vi "test_F9P.vi"() -> ()   [LabVIEW 2019] (continued)
3*05\r\n$GNGSA,A,3,28,11,14,13,33,08,10,,,,,,1.09,0.62,0.90,4*05\r\n$GPGSV,4,1,13,02,65,334,46,04,08,037,34,05,48,261,21,06,58,076,43,1*69\r\n$GPGSV,4,2,13,07,06,105,26,09,38,057,45,12,18,263,29,13,08,191,21,1*66\r\n$GPGSV,4,3,13,17,19,158,23,19,37,161,24,25,11,294,,29,07,323,20,1*6A\r\n$GPGSV,4,4,13,30,01,134,,1*52\r\n$GPGSV,4,1,13,02,65,334,,04,08,037,19,05,48,261,30,06,58,076,31,6*66\r\n$GPGSV,4,2,13,07,06,105,,09,38,057,39,12,18,263,,13,08,191,,6*66\r\n$GPGSV,4,3,13,17,19,158,24,19,37,161,,25,11,294,,29,07,323,,6*6E\r\n$GPGSV,4,4,13,30,01,134,,6*55\r\n$GLGSV,2,1,06,70,54,030,36,71,69,224,32,72,18,217,37,84,08,134,09,1*76\r\n$GLGSV,2,2,06,85,63,113,40,86,52,337,,1*7F\r\n$GLGSV,2,1,06,70,54,030,,71,69,224,17,72,18,217,26,84,08,134,15,3*7B\r\n$GLGSV,2,2,06,85,63,113,24,86,52,337,,3*7F\r\n$GAGSV,3,1,09,02,04,287,07,04,68,085,40,09,44,196,29,11,78,037,39,7*7A\r\n$GAGSV,3,2,09,12,32,115,31,18,55,284,29,19,17,042,20,25,01,241,,7*79\r\n$GAGSV,3,3,09,36,35,314,37,7*4B\r\n$GAGSV,3,1,09,02,04,287,,04,68,085,36,09,44,196,33,11,78,037,28,2*72\r\n$GAGSV,3,2,09,12,32,115,27,18,55,284,38,19,17,042,33,25,01,241,,2*79\r\n$GAGSV,3,3,09,36,35,314,23,2*4B\r\n$GBGSV,4,1,13,04,35,133,,05,09,257,,06,27,182,,07,09,201,,1*7B\r\n$GBGSV,4,2,13,08,65,355,41,09,07,194,,10,16,222,18,11,37,142,22,1*73\r\n$GBGSV,4,3,13,13,50,315,42,14,76,037,41,28,59,310,42,33,73,239,15,1*7A\r\n$GBGSV,4,4,13,34,13,142,17,1*40\r\n$GBGSV,4,1,13,04,35,133,,05,09,257,,06,27,182,,07,09,201,16,3*7E\r\n$GBGSV,4,2,13,08,65,355,35,09,07,194,,10,16,222,27,11,37,142,32,3*7F\r\n$GBGSV,4,3,13,13,50,315,40,14,76,037,28,28,59,310,,33,73,239,,3*77\r\n$GBGSV,4,4,13,34,13,142,,3*44\r\n$GNGLL,3723.61676,N,12656.96910,E,064321.00,A,A*71\r\n$GNRMC,064322.00,A,3723.61692,N,12656.96920,E,0.256,,250720,,,A,V*1B\r\n$GNVTG,,T,,M,0.256,N,0.474,K,A*3B\r\n$GNGGA,064322.00,3723.61692,N,12656.96920,E,1,12,0.62,44.9,M,18.5,M,,*7C\r\n$GNGSA,A,3,17,19,06,05,02,12,09,,,,,,1.07,0.62,0.87,1*09\r\n$GNGSA,A,3,85,70,71,72,,,,,,,,,1.07,0.62,0.87,2*06\r\n$GNGSA,A,3,36,19,11,04,09,12,,,,,,,1.07,0.62,0.87,3*0D\r\n$GNGSA,A,3,28,14,13,33,08,10,,,,,,,1.07,0.62,0.87,4*0D\r\n$GPGSV,4,1,13,02,65,334,45,04,08,037,35,05,48,261,30,06,58,076,44,1*6C\r\n$GPGSV,4,2,13,07,06,105,25,09,38,057,44,12,18,263,28,13,08,191,20,1*64\r\n$GPGSV,4,3,13,17,19,158,30,19,37,161,31,25,11,294,,29,07,323,20,1*6C\r\n$GPGSV,4,4,13,30,01,134,,1*52\r\n$GPGSV,4,1,13,02,65,334,,04,08,037,19,05,48,261,34,06,58,076,33,6*60\r\n$GPGSV,4,2,13,07,06,105,,09,38,057,41,12,18,263,,13,08,191,,6*69\r\n$GPGSV,4,3,13,17,19,158,24,19,37,161,,25,11,294,,29,07,323,,6*6E\r\n$GPGSV,4,4,13,30,01,134,,6*55\r\n$GLGSV,2,1,06,70,54,030,36,71,69,224,31,72,18,217,41,84,08,134,12,1*7E\r\n$GLGSV,2,2,06,85,63,113,39,86,52,337,,1*71\r\n$GLGSV,2,1,06,70,54,030,,71,69,224,17,72,18,217,26,84,08,134,18,3*76\r\n$GLGSV,2,2,06,85,63,113,23,86,52,337,,3*78\r\n$GAGSV,3,1,09,02,04,287,09,04,68,085,41,09,44,196,36,11,78,037,39,7*7B\r\n$GAGSV,3,2,09,12,32,115,35,18,55,284,24,19,17,042,30,25,01,241,,7*71\r\n$GAGSV,3,3,09,36,35,314,35,7*49\r\n$GAGSV,3,1,09,02,04,287,,04,68,085,36,09,44,196,33,11,78,037,28,2*72\r\n$GAGSV,3,2,09,12,32,115,27,18,55,284,37,19,17,042,28,25,01,241,,2*7C\r\n$GAGSV,3,3,09,36,35,314,23,2*4B\r\n$GBGSV,4,1,13,04,35,133,,05,09,257,,06,27,182,,07,09,201,,1*7B\r\n$GBGSV,4,2,13,08,65,355,41,09,07,194,,10,16,222,17,11,37,142,24,1*7A\r\n$GBGSV,4,3,13,13,50,315,42,14,76,037,41,28,59,310,42,33,73,239,27,1*7B\r\n$GBGSV,4,4,13,34,13,142,17,1*40\r\n$GBGSV,4,1,13,04,35,133,,05,09,257,,06,27,182,,07,09,201,16,3*7E\r\n$GBGSV,4,2,13,08,65,355,31,09,07,194,,10,16,222,27,11,37,142,,3*7A\r\n$GBGSV,4,3,13,13,50,315,40,14,76,037,36,28,59,310,,33,73,239,,3*78\r\n$GBGSV,4,4,13,34,13,142,,3*44\r\n$GNGLL,3723.61692,N,12656.96920,E,064322.00,A,A*7B\r\n$GNRMC,064323.00,A,3723.61711,N,12656.96949,E,1.226,107.58,250720,,,A,V*0C\r\n$GNVTG,107.58,T,,M,1.226,N,2.271,K,A*29\r\n$GNGGA,064323.00,3723.61711,N,12656.96949,E,1,12,0.62,44.9,M,18.5,M,,*78\r\n$GNGSA,A,3,17,19,06,05,02,12,09,,,,,,1.09,0.62,0.90,1*01\r\n$GNGSA,A,3,85,70,71,72,,,,,,,,,1.09,0.62,0.90,2*0E\r\n$GNGSA,A,3,36,19,11,04,09,12,,,,,,,1.09,0.62,0.90,3*05\r\n$GNGSA,A,3,28,11,14,13,33,08,10,,,,,,1.09,0.62,0.90,4*05\r\n$GPGSV,4,1,13,02,65,334,44,04,08,037,37,05,48,261,36,06,58,076,46,1*6B\r\n$GPGSV,4,2,13,07,06,105,24,09,38,057,44,12,18,263,27,13,08,191,18,1*61\r\n$GPGSV,4,3,13,17,19,158,29,19,37,161,30,25,11,294,,29,07,323,19,1*6F\r\n$GPGSV,4,4,13,30,01,134,,1*52\r\n$GPGSV,4,1,13,02,65,334,,04,08,037,28,05,48,261,35,06,58,076,36,6*66\r\n$GPGSV,4,2,13,07,06,105,,09,38,057,38,12,18,263,,13,08,191,,6*67\r\n$GPGSV,4,3,13,17,19,158,22,19,37,161,,25,11,294,,29,07,323,,6*68\r\n$GPGSV,4,4,13,30,01,134,,6*55\r\n$GLGSV,2,1,06,70,54,030,33,71,69,224,33,72,18,217,38,84,08,134,11,1*74\r\n$GLGSV,2,2,06,85,63,113,35,86,52,337,,1*7D\r\n$GLGSV,2,1,06,70,54,030,,71,69,224,18,72,18,217,26,84,08,134,15,3*74\r\n$GLGSV,2,2,06,85,63,113,22,86,52,337,,3*79\r\n$GAGSV,3,1,09,02,04,287,12,04,68,085,38,09,44,196,32,11,78,037,37,7*75\r\n$GAGSV,3,2,09,12,32,115,32,18,55,284,26,19,17,042,34,25,01,241,,7*70\r\n$GAGSV,3,3,09,36,35,314,27,7*4A\r\n$GAGSV,3,1,09,02,04,287,,04,68,085,31,09,44,196,32,11,78,037,33,2*7E\r\n$GAGSV,3,2,09,12,32,115,33,18,55,284,35,19,17,042,32,25,01,241,,2*70\r\n$GAGSV,3,3,09,36,35,314,23,2*4B\r\n$GBGSV,4,1,13,04,35,133,,05,09,257,,06,27,182,,07,09,201,,1*7B\r\n$GBGSV,4,2,13,08,65,355,41,09,07,194,,10,16,222,15,11,37,142,31,1*7C\r\n$GBGSV,4,3,13,13,50,315,42,14,76,037,42,28,59,310,44,33,73,239,35,1*7D\r\n$GBGSV,4,4,13,34,13,142,20,1*44\r\n$GBGSV,4,1,13,04,35,133,,05,09,257,,06,27,182,,07,09,201,17,3*7F\r\n$GBGSV,4,2,13,08,65,355,34,09,07,194,,10,16,222,24,11,37,142,,3*7C\r\n$GBGSV,4,3,13,13,50,315,41,14,76,037,41,28,59,310,,33,73,239,,3*79\r\n$GBGSV,4,4,13,34,13,142,,3*44\r\n$GNGLL,3723.61711,N,12656.96949,E,064323.00,A,A*7F\r\n$GNRMC,064324.00,A,3723.61742,N,12656.97004,E,2.052,73.76,250720,,,A,V*30\r\n$GNVTG,73.76,T,,M,2.052,N,3.800,K,A*18\r\n$GNGGA,064324.00,3723.61742,N,12656.97004,E,1,12,0.66,44.7,M,18.5,M,,*72\r\n$GNGSA,A,3,17,19,06,05,02,09,,,,,,,1.18,0.66,0.98,1*0E\r\n$GNGSA,A,3,85,70,71,72,,,,,,,,,1.18,0.66,0.98,2*02\r\n$GNGSA,A,3,36,19,11,04,09,12,,,,,,,1.18,0.66,0.98,3*09\r\n$GNGSA,A,3,28,11,14,13,34,33,08,10,,,,,1.18,0.66,0.98,4*0E\r\n$GPGSV,4,1,13,02,65,334,46,04,08,037,37,05,48,261,37,06,58,076,37,1*6E\r\n$GPGSV,4,2,13,07,06,105,31,09,38,057,43,12,18,263,,13,08,191,,1*6E\r\n$GPGSV,4,3,13,17,19,158,22,19,37,161,34,25,11,294,25,29,07,323,18,1*66\r\n$GPGSV,4,4,13,30,01,134,,1*52\r\n$GPGSV,4,1,13,02,65,334,,04,08,037,38,05,48,261,36,06,58,076,37,6*65\r\n$GPGSV,4,2,13,07,06,105,,09,38,057,41,12,18,263,,13,08,191,,6*69\r\n$GPGSV,4,3,13,17,19,158,20,19,37,161,,25,11,294,,29,07,323,,6*6A\r\n$GPGSV,4,4,13,30,01,134,,6*55\r\n$GLGSV,2,1,06,70,54,030,38,71,69,224,37,72,18,217,34,84,08,134,12,1*74\r\n$GLGSV,2,2,06,85,63,113,29,86,52,337,,1*70\r\n$GLGSV,2,1,06,70,54,030,,71,69,224,32,72,18,217,27,84,08,134,14,3*7C\r\n$GLGSV,2,2,06,85,63,113,30,86,52,337,,3*7A\r\n$GAGSV,3,1,09,02,04,287,11,04,68,085,35,09,44,196,26,11,78,037,39,7*70\r\n$GAGSV,3,2,09,12,32,115,28,18,55,284,37,19,17,042,35,25,01,241,,7*7A\r\n$GAGSV,3,3,09,36,35,314,26,7*4B\r\n$GAGSV,3,1,09,02,04,287,,04,68,085,32,09,44,196,26,11,78,037,27,2*7D\r\n$GAGSV,3,2,09,12,32,115,29,18,55,284,38,19,17,042,36,25,01,241,,2*72\r\n$GAGSV,3,3,09,36,35,314,23,2*4B\r\n$GBGSV,4,1,13,04,35,133,,05,09,257,,06,27,182,,07,09,201,,1*7B\r\n$GBGSV,4,2,13,08,65,355,42,09,07,194,,10,16,222,15,11,37,142,32,1*7C\r\n$GBGSV,4,3,13,13,50,315,43,14,76,037,42,28,59,310,43,33,73,239,39,1*77\r\n$GBGSV,4,4,13,34,13,142,22,1*46\r\n$GBGSV,4,1,13,04,35,133,,05,09,257,,06,27,182,,07,09,201,19,3*71\r\n$GBGSV,4,2,13,08,65,355,36,09,07,194,,10,16,222,21,11,37,142,,3*7B\r\n$GBGSV,4,3,13,13,50,315,39,14,76,037,33,28,59,310,,33,73,239,,3*73\r\n$GBGSV,4,4,13,34,13,142,,3*44\r\n$GNGLL,3723.61742,N,12656.97004,E,064324.00,A,A*7F\r\n$GNRMC,064325.00,A,3723.61775,N,12656.97077,E,2.478,66.36,250720,,,A,V*3D\r\n$GNVTG,66.36,T,,M,2.478,N,4.589,K,A*1F\r\n$GNGGA,064325.00,3723.61775,N,12656.97077,E,1,12,0.66,44.5,M,18.5,M,,*71\r\n$GNGSA,A,3,17,19,06,05,02,09,,,,,,,1.18,0.66,0.98,1*0E\r\n$GNGSA,A,3,85,70,71,72,,,,,,,,,1.18,0.66,0.98,2*02\r\n$GNGSA,A,3,36,19,11,04,09,12,,,,,,,1.18,0.66,0.98,3*09\r\n$GNGSA,A,3,28,11,14,13,33,08,10,,,,,,1.18,0.66,0.98,4*09\r\n$GPGSV,4,1,13,02,66,335,48,04,08,037,36,05,48,261,33,06,58,076,42,1*65\r\n$GPGSV,4,2,13,07,06,105,,09,38,057,45,12,18,263,,13,08,191,,1*6A\r\n$GPGSV,4,3,13,17,19,158,25,19,37,161,36,25,11,294,22,29,07,323,18,1*64\r\n$GPGSV,4,4,13,30,01,134,,1*52\r\n$GPGSV,4,1,13,02,66,335,,04,08,037,40,05,48,261,38,06,58,076,36,6*67\r\n$GPGSV,4,2,13,07,06,105,,09,38,057,35,12,18,263,22,13,08,191,,6*6A\r\n$GPGSV,4,3,13,17,19,158,20,19,37,161,,25,11,294,,29,07,323,,6*6A\r\n$GPGSV,4,4,13,30,01,134,,6*55\r\n$GLGSV,2,1,06,70,54,030,39,71,69,224,35,72,18,217,32,84,08,134,09,1*7B\r\n$GLGSV,2,2,06,85,63,113,34,86,52,337,,1*7C\r\n$GLGSV,2,1,06,70,54,030,,71,69,224,26,72,18,217,27,84,08,134,15,3*78\r\n$GLGSV,2,2,06,85,63,113,28,86,52,337,,3*73\r\n$GAGSV,3,1,09,02,04,287,09,04,68,085,36,09,44,196,32,11,78,037,39,7*7F\r\n$GAGSV,3,2,09,12,32,115,32,18,55,284,36,19,17,042,35,25,01,241,,7*70\r\n$GAGSV,3,3,09,36,35,314,26,7*4B\r\n$GAGSV,3,1,09,02,04,287,,04,68,085,31,09,44,196,26,11,78,037,32,2*7A\r\n$GAGSV,3,2,09,12,32,115,28,18,55,284,39,19,17,042,36,25,01,241,,2*72\r\n$GAGSV,3,3,09,36,35,314,22,2*4A\r\n$GBGSV,4,1,13,04,35,133,,05,09,257,,06,27,182,,07,09,201,,1*7B\r\n$GBGSV,4,2,13,08,65,355,41,09,07,194,,10,16,222,15,11,37,142,27,1*7B\r\n$GBGSV,4,3,13,13,50,315,45,14,76,037,41,28,59,310,44,33,73,239,38,1*74\r\n$GBGSV,4,4,13,34,13,142,,1*46\r\n$GBGSV,4,1,13,04,35,133,,05,09,257,,06,27,182,,07,09,201,20,3*7B\r\n$GBGSV,4,2,13,08,65,355,38,09,07,194,,10,16,222,18,11,37,142,,3*7F\r\n$GBGSV,4,3,13,13,50,315,40,14,76,037,34,28,59,310,,33,73,239,,3*7A\r\n$GBGSV,4,4,13,34,13,142,,3*44\r\n$GNGLL,3723.61775,N,12656.97077,E,064325.00,A,A*7E\r\n$GNRMC,064326.00,A,3723.61798,N,12656.97166,E,2.758,70.76,250720,,,A,V*3E\r\n$GNVTG,70.76,T,,M,2.758,N,5.109,K,A*10\r\n$GNGGA,064326.00,3723.61798,N,12656.97166,E,1,12,0.66,44.4,M,18.5,M,,*71\r\n$GNGSA,A,3,17,19,06,05,02,09,,,,,,,1.18,0.66,0.98,1*0E\r\n$GNGSA,A,3,85,70,71,72,,,,,,,,,1.18,0.66,0.98,2*02\r\n$GNGSA,A,3,36,19,11,04,09,12,,,,,,,1.18,0.66,0.98,3*09\r\n$GNGSA,A,3,28,11,14,13,33,08,10,,,,,,1.18,0.66,0.98,4*09\r\n$GPGSV,4,1,13,02,66,335,46,04,08,037,42,05,48,261,36,06,58,076,43,1*6C\r\n$GPGSV,4,2,13,07,06,105,,09,38,057,44,12,18,263,23,13,08,191,25,1*6D\r\n$GPGSV,4,3,13,17,19,158,25,19,37,161,36,25,11,294,20,29,07,323,19,1*67\r\n$GPGSV,4,4,13,30,01,134,,1*52\r\n$GPGSV,4,1,13,02,66,335,,04,08,037,39,05,48,261,40,06,58,076,35,6*65\r\n$GPGSV,4,2,13,07,06,105,,09,38,057,38,12,18,263,19,13,08,191,,6*6F\r\n$GPGSV,4,3,13,17,19,158,28,19,37,161,,25,11,294,,29,07,323,,6*62\r\n$GPGSV,4,4,13,30,01,134,,6*55\r\n$GLGSV,2,1,06,70,54,030,34,71,69,224,39,72,18,217,32,84,08,134,12,1*70\r\n$GLGSV,2,2,06,85,63,113,35,86,52,337,,1*7D\r\n$GLGSV,2,1,06,70,54,030,,71,69,224,26,72,18,217,25,84,08,134,16,3*79\r\n$GLGSV,2,2,06,85,63,113,27,86,52,337,,3*7C\r\n$GAGSV,3,1,09,02,04,287,12,04,68,085,41,09,44,196,26,11,78,037,39,7*70\r\n$GAGSV,3,2,09,12,32,115,28,18,55,284,39,19,17,042,35,25,01,241,,7*74\r\n$GAGSV,3,3,09,36,35,314,25,7*48\r\n$GAGSV,3,1,09,02,04,287,,04,68,085,32,09,44,196,23,11,78,037,32,2*7C\r\n$GAGSV,3,2,09,12,32,115,33,18,55,284,37,19,17,042,28,25,01,241,,2*79\r\n$GAGSV,3,3,09,36,35,314,21,2*49\r\n$GBGSV,4,1,13,04,35,133,,05,09,257,,06,27,182,,07,09,201,,1*7B\r\n$GBGSV,4,2,13,08,65,355,42,09,07,194,,10,16,222,17,11,37,142,31,1*7D\r\n$GBGSV,4,3,13,13,50,315,45,14,76,037,44,28,59,310,36,33,73,239,42,1*79\r\n$GBGSV,4,4,13,34,13,142,,1*46\r\n$GBGSV,4,1,13,04,35,133,,05,09,257,,06,27,182,,07,09,201,21,3*7A\r\n$GBGSV,4,2,13,08,65,355,38,09,07,194,,10,16,222,20,11,37,142,,3*74\r\n$GBGSV,4,3,13,13,50,315,40,14,76,037,38,28,59,310,,33,73,239,,3*76\r\n$GBGSV,4,4,13,34,13,142,,3*44\r\n$GNGLL,3723.61798,N,12656.97166,E,064326.00,A,A*7F\r\n$GNRMC,064327.00,A,3723.61827,N,12656.97258,E,2.933,66.94,250720,,,A,V*32\r\n$GNVTG,66.94,T,,M,2.933,N,5.432,K,A*15\r\n$GNGGA,064327.00,3723.61827,N,12656.97258,E,1,12,0.66,44.5,M,18.5,M,,*74\r\n$GNGSA,A,3,17,19,06,05,02,09,,,,,,,1.18,0.66,0.98,1*0E\r\n$GNGSA,A,3,85,70,71,72,,,,,,,,,1.18,0.66,0.98,2*02\r\n$GNGSA,A,3,36,19,11,04,09,12,,,,,,,1.18,0.66,0.98,3*09\r\n$GNGSA,A,3,28,11,14,13,33,34,08,10,,,,,1.18,0.66,0.98,4*0E\r\n$GPGSV,4,1,13,02,66,335,42,04,08,037,42,05,48,261,41,06,58,076,44,1*6F\r\n$GPGSV,4,2,13,07,06,105,,09,38,057,48,12,18,263,,13,08,191,25,1*60\r\n$GPGSV,4,3,13,17,19,158,27,19,37,161,32,25,11,294,18,29,07,323,17,1*64\r\n$GPGSV,4,4,13,30,01,134,,1*52\r\n$GPGSV,4,1,13,02,66,335,,04,08,037,35,05,48,261,37,06,58,076,37,6*6B\r\n$GPGSV,4,2,13,07,06,105,,09,38,057,40,12,18,263,13,13,08,191,,6*6A\r\n$GPGSV,4,3,13,17,19,158,25,19,37,161,,25,11,294,,29,07,323,,6*6F\r\n$GPGSV,4,4,13,30,01,134,,6*55\r\n$GLGSV,2,1,06,70,54,030,31,71,69,224,40,72,18,217,32,84,08,134,14,1*7D\r\n$GLGSV,2,2,06,85,63,113,33,86,52,337,,1*7B\r\n$GLGSV,2,1,06,70,54,030,,71,69,224,26,72,18,217,23,84,08,134,14,3*7D\r\n$GLGSV,2,2,06,85,63,113,26,86,52,337,,3*7D\r\n$GAGSV,3,1,09,02,04,287,08,04,68,085,43,09,44,196,27,11,78,037,39,7*78\r\n$GAGSV,3,2,09,12,32,115,28,18,55,284,38,19,17,042,37,25,01,241,,7*77\r\n$GAGSV,3,3,09,36,35,314,31,7*4D\r\n$GAGSV,3,1,09,02,04,287,,04,68,085,36,09,44,196,22,11,78,037,32,2*79\r\n$GAGSV,3,2,09,12,32,115,28,18,55,284,42,19,17,042,38,25,01,241,,2*70\r\n$GAGSV,3,3,09,36,35,314,23,2*4B\r\n$GBGSV,4,1,13,04,35,133,,05,09,257,,06,27,182,,07,09,201,,1*7B\r\n$GBGSV,4,2,13,08,65,355,42,09,07,194,,10,16,222,17,11,37,142,27,1*7A\r\n$GBGSV,4,3,13,13,50,315,37,14,76,037,44,28,59,310,42,33,73,239,40,1*7D\r\n$GBGSV,4,4,13,34,13,142,33,1*46\r\n$GBGSV,4,1,13,04,35,133,,05,09,257,,06,27,182,,07,09,201,23,3*78\r\n$GBGSV,4,2,13,08,65,355,36,09,07,194,,10,16,222,21,11,37,142,,3*7B\r\n$GBGSV,4,3,13,13,50,315,34,14,76,037,35,28,59,310,,33,73,239,,3*78\r\n$GBGSV,4,4,13,34,13,142,,3*44\r\n$GNGLL,3723.61827,N,12656.97258,E,064327.00,A,A*7B\r\n$GNRMC,064328.00,A,3723.61847,N,12656.97349,E,2.893,70.77,250720,,,A,V*3B\r\n$GNVTG,70.77,T,,M,2.893,N,5.358,K,A*1F\r\n$GNGGA,064328.00,3723.61847,N,12656.97349,E,1,12,0.66,44.2,M,18.5,M,,*7B\r\n$GNGSA,A,3,17,19,06,05,02,09,,,,,,,1.18,0.66,0.98,1*0E\r\n$GNGSA,A,3,85,70,71,72,,,,,,,,,1.18,0.66,0.98,2*02\r\n$GNGSA,A,3,36,19,11,04,09,12,,,,,,,1.18,0.66,0.98,3*09\r\n$GNGSA,A,3,28,11,14,13,33,08,10,,,,,,1.18,0.66,0.98,4*09\r\n$GPGSV,4,1,13,02,66,335,45,04,08,037,38,05,48,262,42,06,58,076,43,1*62\r\n$GPGSV,4,2,13,07,06,105,,09,38,057,47,12,18,263,,13,08,191,,1*68\r\n$GPGSV,4,3,13,17,19,158,31,19,37,161,28,25,11,294,18,29,07,323,17,1*68\r\n$GPGSV,4,4,13,30,01,134,,1*52\r\n$GPGSV,4,1,13,02,66,335,,04,08,037,36,05,48,262,39,06,58,076,33,6*61\r\n$GPGSV,4,2,13,07,06,105,,09,38,057,41,12,18,263,12,13,08,191,,6*6A\r\n$GPGSV,4,3,13,17,19,158,25,19,37,161,,25,11,294,,29,07,323,,6*6F\r\n$GPGSV,4,4,13,30,01,134,,6*55\r\n$GLGSV,2,1,06,70,54,030,35,71,69,224,39,72,18,217,27,84,08,134,11,1*76\r\n$GLGSV,2,2,06,85,63,113,35,86,52,337,,1*7D\r\n$GLGSV,2,1,06,70,54,030,,71,69,224,27,72,18,217,21,84,08,134,14,3*7E\r\n$GLGSV,2,2,06,85,63,113,27,86,52,337,,3*7C\r\n$GAGSV,3,1,09,02,04,287,10,04,68,085,41,09,44,196,26,11,78,037,39,7*72\r\n$GAGSV,3,2,09,12,32,115,29,18,55,284,39,19,17,042,42,25,01,241,,7*75\r\n$GAGSV,3,3,09,36,35,314,25,7*48\r\n$GAGSV,3,1,09,02,04,287,,04,68,085,33,09,44,196,22,11,78,037,31,2*7F\r\n$GAGSV,3,2,09,12,32,115,27,18,55,284,40,19,17,042,37,25,01,241,,2*72\r\n$GAGSV,3,3,09,36,35,314,24,2*4C\r\n$GBGSV,4,1,13,04,35,133,,05,09,257,,06,27,182,,07,09,201,,1*7B\r\n$GBGSV,4,2,13,08,65,355,42,09,07,194,,10,16,222,18,11,37,142,28,1*7A\r\n$GBGSV,4,3,13,13,50,315,37,14,76,037,42,28,59,310,41,33,73,239,40,1*78\r\n$GBGSV,4,4,13,34,13,142,,1*46\r\n$GBGSV,4,1,13,04,35,133,,05,09,257,,06,27,182,,07,09,201,21,3*7A\r\n$GBGSV,4,2,13,08,65,355,37,09,07,194,,10,16,222,19,11,37,142,,3*71\r\n$GBGSV,4,3,13,13,50,315,35,14,76,037,35,28,59,310,,33,73,239,,3*79\r\n$GBGSV,4,4,13,34,13,142,,3*44\r\n$GNGLL,3723.61847,N,12656.97349,E,064328.00,A,A*73\r\n$GNRMC,064329.00,A,3723.61852,N,12656.97443,E,2.831,76.66,250720,,,A,V*3D\r\n$GNVTG,76.66,T,,M,2.831,N,5.243,K,A*1A\r\n$GNGGA,064329.00,3723.61852,N,12656.97443,E,1,12,0.67,44.0,M,18.5,M,,*70\r\n$GNGSA,A,3,17,19,06,05,02,09,,,,,,,1.19,0.67,0.98,1*0E\r\n$GNGSA,A,3,85,70,71,72,,,,,,,,,1.19,0.67,0.98,2*02\r\n$GNGSA,A,3,36,19,11,04,09,12,,,,,,,1.19,0.67,0.98,3*09\r\n$GNGSA,A,3,28,14,13,33,08,10,,,,,,,1.19,0.67,0.98,4*09\r\n$GPGSV,4,1,13,02,66,335,44,04,08,037,31,05,48,262,42,06,58,077,46,1*6E\r\n$GPGSV,4,2,13,07,06,105,,09,38,057,45,12,18,263,,13,08,191,29,1*61\r\n$GPGSV,4,3,13,17,19,158,32,19,37,161,28,25,11,294,20,29,07,323,16,1*61\r\n$GPGSV,4,4,13,30,01,134,,1*52\r\n$GPGSV,4,1,13,02,66,335,,04,08,037,37,05,48,262,36,06,58,077,37,6*6A\r\n$GPGSV,4,2,13,07,06,105,,09,38,057,39,12,18,263,10,13,08,191,,6*67\r\n$GPGSV,4,3,13,17,19,158,29,19,37,161,,25,11,294,,29,07,323,,6*63\r\n$GPGSV,4,4,13,30,01,134,,6*55\r\n$GLGSV,2,1,06,70,54,030,32,71,69,224,39,72,18,217,29,84,08,134,11,1*7F\r\n$GLGSV,2,2,06,85,63,113,35,86,52,337,,1*7D\r\n$GLGSV,2,1,06,70,54,030,,71,69,224,27,72,18,217,22,84,08,134,12,3*7B\r\n$GLGSV,2,2,06,85,63,113,27,86,52,337,,3*7C\r\n$GAGSV,3,1,09,02,04,287,09,04,68,085,43,09,44,196,26,11,78,037,41,7*77\r\n$GAGSV,3,2,09,12,32,115,33,18,55,284,39,19,17,042,42,25,01,241,,7*7E\r\n$GAGSV,3,3,09,36,35,314,24,7*49\r\n$GAGSV,3,1,09,02,04,287,,04,68,085,38,09,44,196,22,11,78,037,31,2*74\r\n$GAGSV,3,2,09,12,32,115,27,18,55,284,43,19,17,042,37,25,01,241,,2*71\r\n$GAGSV,3,3,09,36,35,314,24,2*4C\r\n$GBGSV,4,1,13,04,35,133,,05,09,257,,06,27,182,,07,09,201,,1*7B\r\n$GBGSV,4,2,13,08,65,355,41,09,07,194,,10,16,222,18,11,37,142,,1*73\r\n$GBGSV,4,3,13,13,50,315,38,14,76,037,45,28,59,310,41,33,73,239,40,1*70\r\n$GBGSV,4,4,13,34,13,142,,1*46\r\n$GBGSV,4,1,13,04,35,133,,05,09,257,,06,27,182,,07,09,201,21,3*7A\r\n$GBGSV,4,2,13,08,65,355,37,09,07,194,,10,16,222,20,11,37,142,,3*7B\r\n$GBGSV,4,3,13,13,50,315,37,14,76,037,37,28,59,310,,33,73,239,,3*79\r\n$GBGSV,4,4,13,34,13,142,,3*44\r\n$GNGLL,3723.61852,N,12656.97443,E,064329.00,A,A*7B\r\n$GNRMC,064330.00,A,3723.61864,N,12656.97538,E,2.885,74.64,250720,,,A,V*32\r\n$GNVTG,74.64,T,,M,2.885,N,5.343,K,A*14\r\n$GNGGA,064330.00,3723.61864,N,12656.97538,E,1,12,0.67,44.0,M,18.5,M,,*70\r\n$GNGSA,A,3,17,19,06,12,05,02,09,,,,,,1.19,0.67,0.98,1*0D\r\n$GNGSA,A,3,85,70,71,72,,,,,,,,,1.19,0.67,0.98,2*02\r\n$GNGSA,A,3,36,19,11,04,09,12,,,,,,,1.19,0.67,0.98,3*09\r\n$GNGSA,A,3,28,14,13,33,08,10,,,,,,,1.19,0.67,0.98,4*09\r\n$GPGSV,4,1,13,02,66,335,42,04,08,037,37,05,48,262,41,06,58,077,45,1*6E\r\n$GPGSV,4,2,13,07,06,104,,09,38,057,44,12,18,263,,13,08,191,20,1*68\r\n$GPGSV,4,3,13,17,19,158,32,19,37,161,35,25,11,294,20,29,07,323,16,1*6D\r\n$GPGSV,4,4,13,30,01,134,,1*52\r\n$GPGSV,4,1,13,02,66,335,,04,08,037,34,05,48,262,38,06,58,077,39,6*69\r\n$GPGSV,4,2,13,07,06,104,,09,38,057,41,12,18,263,11,13,08,191,,6*68\r\n$GPGSV,4,3,13,17,19,158,28,19,37,161,,25,11,294,,29,07,323,,6*62\r\n$GPGSV,4,4,13,30,01,134,,6*55\r\n$GLGSV,2,1,06,70,54,030,31,71,69,224,39,72,18,217,29,84,08,134,08,1*74\r\n$GLGSV,2,2,06,85,63,113,38,86,52,337,,1*70\r\n$GLGSV,2,1,06,70,54,030,,71,69,224,27,72,18,217,21,84,08,134,13,3*79\r\n$GLGSV,2,2,06,85,63,113,27,86,52,337,,3*7C\r\n$GAGSV,3,1,09,02,04,287,12,04,68,085,45,09,44,196,31,11,78,037,41,7*7D\r\n$GAGSV,3,2,09,12,32,115,29,18,55,284,36,19,17,042,34,25,01,241,,7*7B\r\n$GAGSV,3,3,09,36,35,314,24,7*49\r\n$GAGSV,3,1,09,02,04,287,,04,68,085,37,09,44,196,23,11,78,037,31,2*7A\r\n$GAGSV,3,2,09,12,32,115,26,18,55,284,45,19,17,042,31,25,01,241,,2*70\r\n$GAGSV,3,3,09,36,35,314,22,2*4A\r\n$GBGSV,4,1,13,04,35,133,,05,09,257,,06,27,182,,07,09,201,,1*7B\r\n$GBGSV,4,2,13,08,65,355,41,09,07,194,,10,16,222,17,11,37,142,,1*7C\r\n$GBGSV,4,3,13,13,50,315,35,14,76,037,45,28,59,310,42,33,73,239,41,1*7F\r\n$GBGSV,4,4,13,34,13,142,24,1*40\r\n$GBGSV,4,1,13,04,35,133,,05,09,257,,06,27,182,,07,09,201,18,3*70\r\n$GBGSV,4
